vi "SetParentCall.vi"(8 "error in (no error)":errorcluster, 10 "Parent Call":T1, 11 "SMO in":refnum<class "SMO.lvclass">) -> (0 "error out":errorcluster, 3 "SMO out":refnum<class "SMO.lvclass">)   [LabVIEW 2013, in "SMO.lvclass"]
uses:
  SMO.lvclass
  Typedefs/Parent Call--Enum.ctl
  SMO.lvclass/SMO.ctl
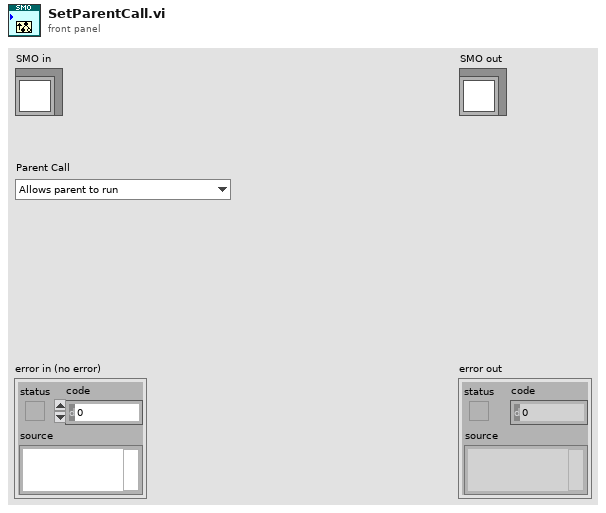
[diagram p1: front panel]
types:
  T1 = typedef "SMO.lvclass/Parent Call--Enum.ctl" = enum16{"Allows parent to run", "Does not request parent to run"}
  T2 = typedef "SMO.lvclass/PrivateData--Ref.ctl" = refnum<data-value>
  T3 = typedef "SMO.lvclass/PrivateData--Cluster.ctl" = cluster{"Parent Call":T1, "Registered Processes":T4[], "Sync Notifier":refnum<notifier>, "Process Error Notifier":refnum<notifier>, "Protected Events":T5, "Public Events":T6, "SMO State":T7, "[Dependencies]":T8[], "[Attributes]":refnum<class "Attribute.lvclass">[], "Launcher Close":refnum<notifier>}
  T4 = typedef "SMO.lvclass/RegisteredProcessData--Cluster.ctl" = cluster{"Name":string, "Static VI Ref":refnum<vi>, "Running":bool, "NotifierRef":u32}
  T5 = typedef "SMO.lvclass/Protected Events.ctl" = cluster{"StopProcesses":refnum<user-event>, "AbortProcesses":refnum<user-event>, "Config Changed":refnum<user-event>}
  T6 = typedef "SMO.lvclass/Public Events.ctl" = cluster{"Error":refnum<user-event>, "State":refnum<user-event>}
  T7 = typedef "SMO.lvclass/SMOState --Enum.ctl" = enum16{"unknown", "Created", "Started", "Stopped"}
  T8 = typedef "SMO.lvclass/SMO Dependency--Cluster.ctl" = cluster{"Dependency":refnum<class "SMO.lvclass">, "Level":string}
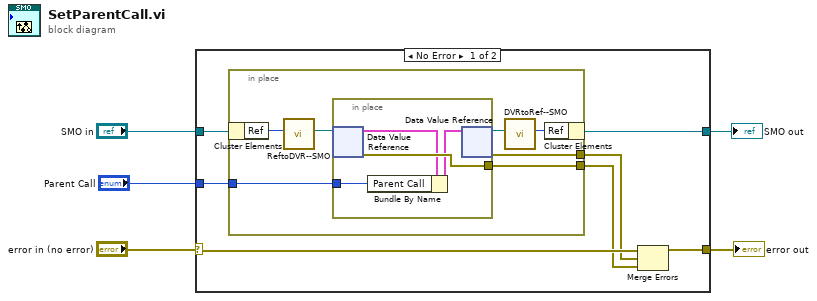
[diagram p0: block diagram]
diagram:
  n1 = case shown="No Error" "error in (no error)" {
    selector: "error in (no error)" -> [w10 w25]
    tunnel: [w9 w25] -> w2
    tunnel: [w11 w24] -> w1
    tunnel: "SMO in" -> [w12 w24]
    tunnel: "Parent Call" -> [w6 _]
    frame No Error {
      n2 = in-place {
        in-place-border: [w19] -> w8
        in-place-border: [w18] -> w7
        in-place-border: w6 -> [w13]
        n3 = in-place-cluster #1(w12) -> ("Ref"=w17:u32)
        n4 = call "ReftoDVR--SMO.vi"("Ref"=w17) -> ("Ref"=w16:T2)  [unwired: 10 in]
        n5 = in-place {
          in-place-border: [w23] -> w18
          in-place-border: w13 -> [w20]
          n6 = in-place-dvr #2(w16) -> (w22:T3, w23:errorcluster)
          n7 = Bundle By Name(cluster=w22, "Parent Call"=w20) -> (w21:T3)
          n8 = in-place-dvr #2(w21) -> (w15:T2, w19:errorcluster)
        }
        n9 = call "DVRtoRef--SMO.vi"("Ref"=w15) -> ("Ref"=w14:u32)  [unwired: 10 in]
        n10 = in-place-cluster #1("Ref"=w14) -> (w11:refnum<class "SMO.lvclass">)
      }
      n11 = Merge Errors(w10, w8, w7) -> (w9:errorcluster)
    }
    frame Error {
    }
  }
  "error out" <- w2
  "SMO out" <- w1
